vi "期末專題-記憶遊戲.vi"() -> ()   [LabVIEW 2014]
uses:
  States.ctl
  Application data.ctl
panel:
  in  "顏色順序按鈕":T1
  out "記住的顏色個數":i32
  out "顏色記憶順序":u32(colorbox)
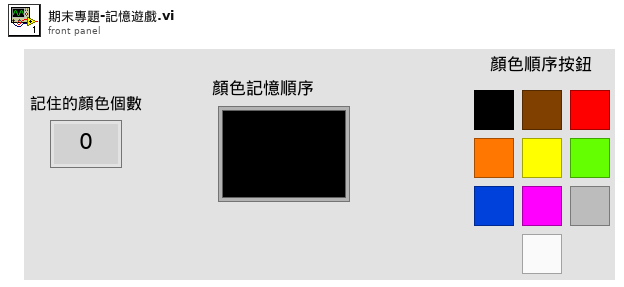
[diagram p1: front panel]
types:
  T1 = cluster{"0":bool, "7":bool, "8":bool, "9":bool, "4":bool, "5":bool, "6":bool, "1":bool, "2":bool, "3":bool}
  T2 = typedef "Application data.ctl" = cluster{"順序":i32[], "顏色":u32[], "等待時間":u32, "Last key":i16, "No.Key presses":i32, "得分":i32}
  T3 = typedef "States.ctl" = enum16{"開始", "加入新顏色", "順序", "等待", "檢查按鈕", "成功", "失敗", "結束"}
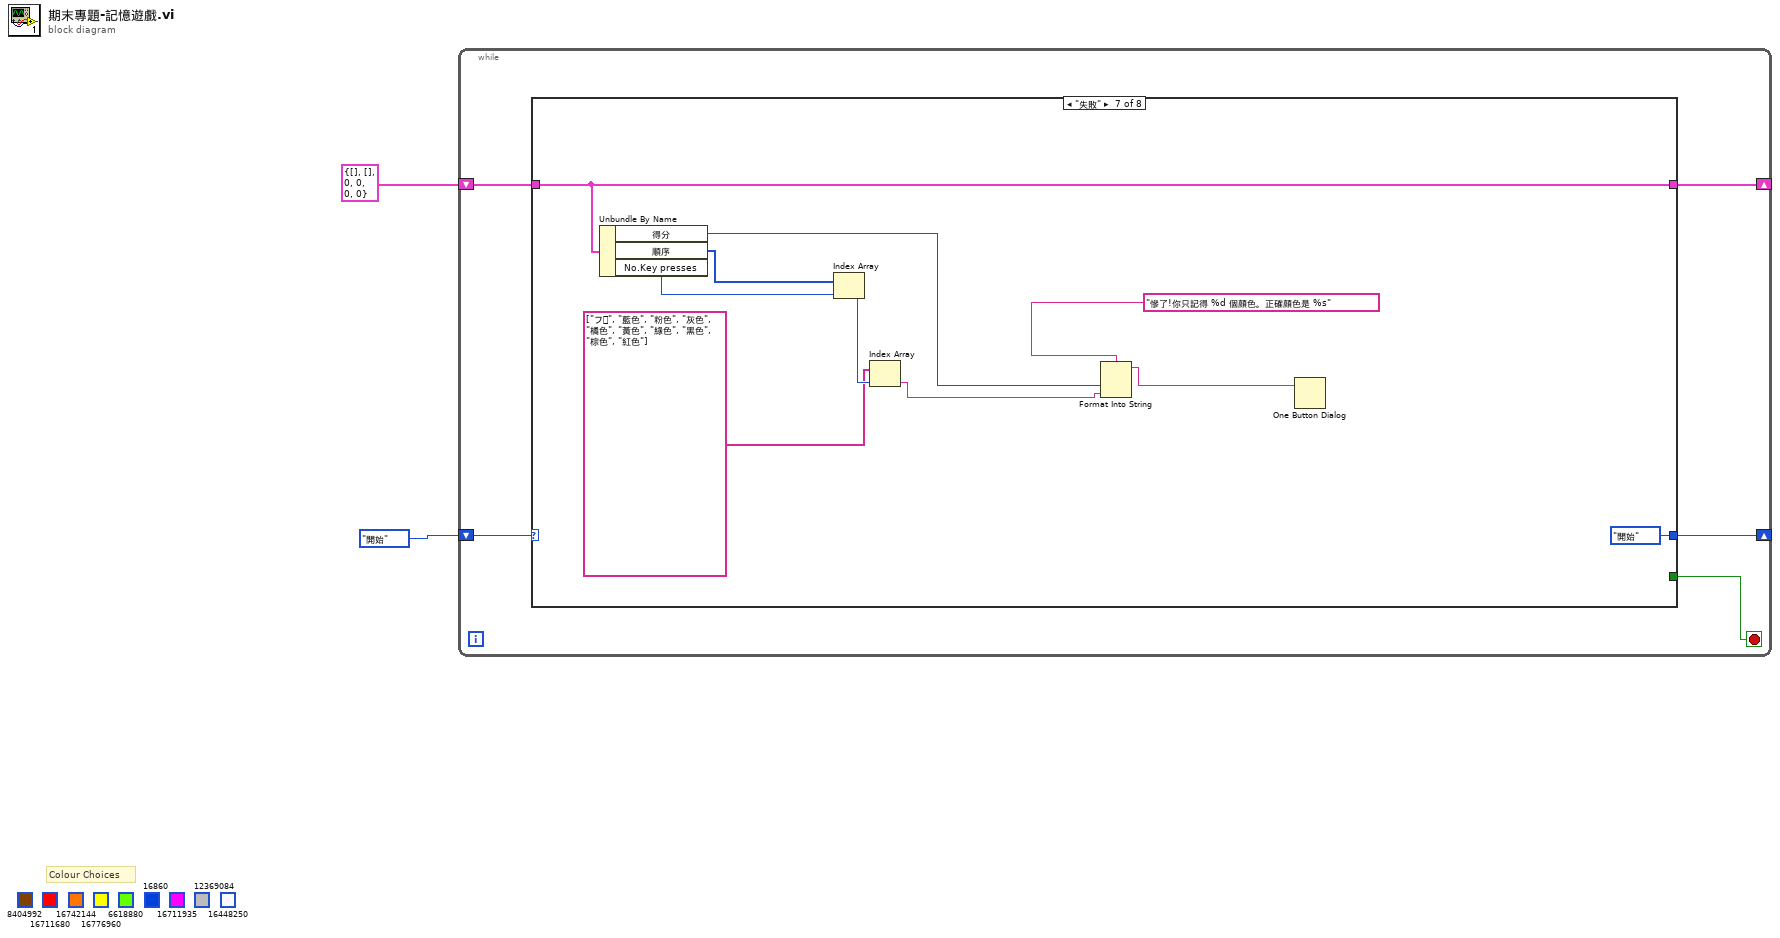
[diagram p0: block diagram]
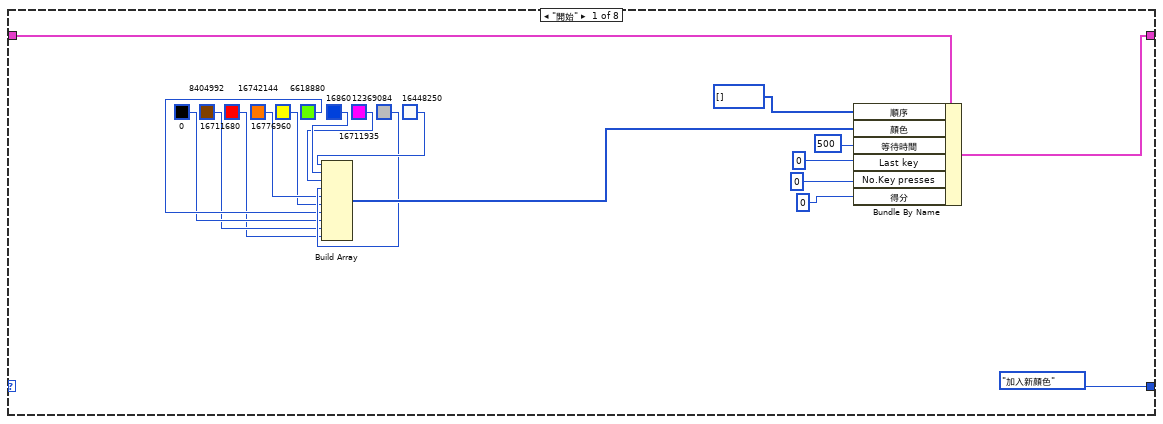
[diagram p2: hidden frame]
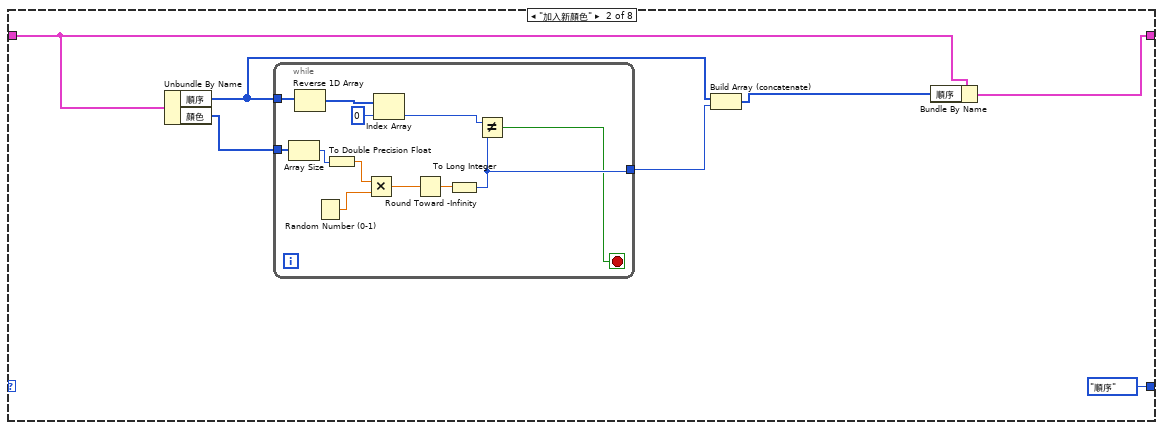
[diagram p3: hidden frame]
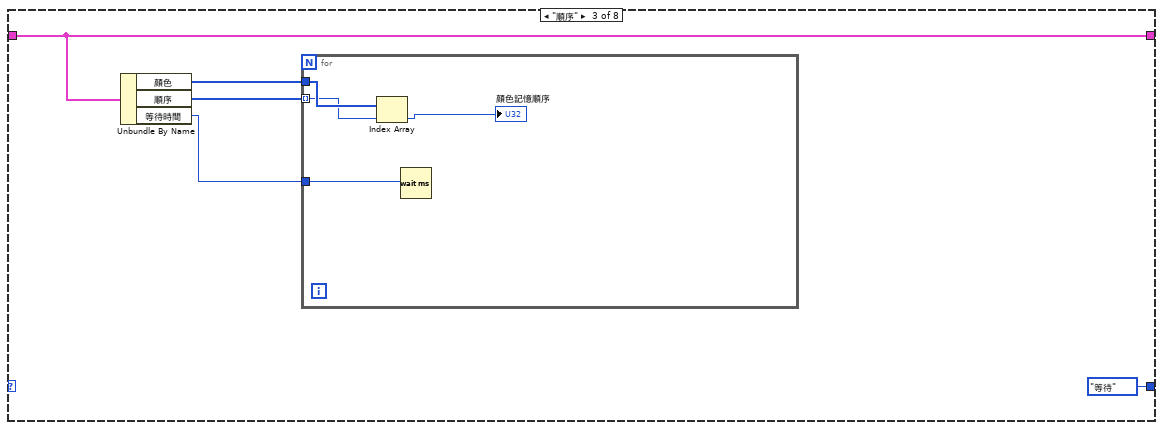
[diagram p4: hidden frame]
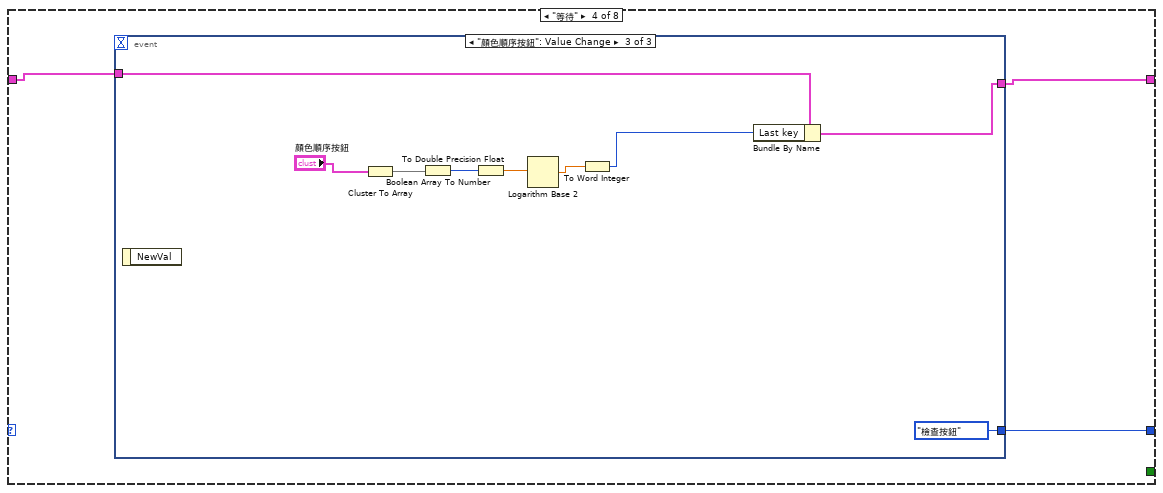
[diagram p5: hidden frame]
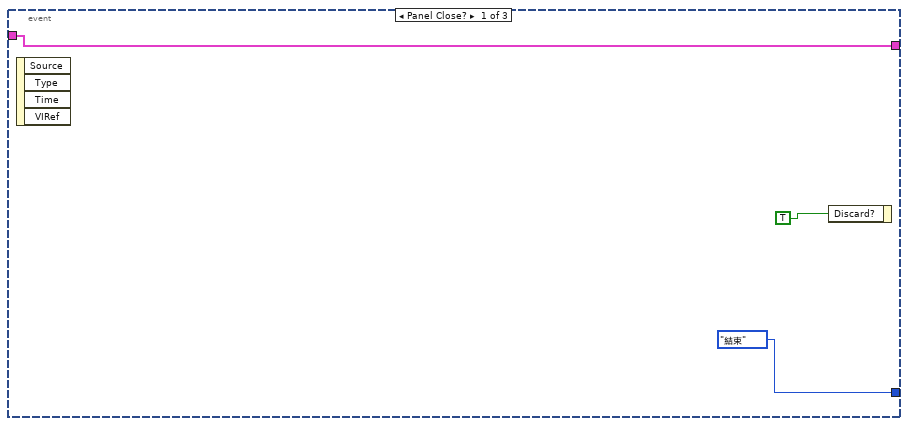
[diagram p6: hidden frame]
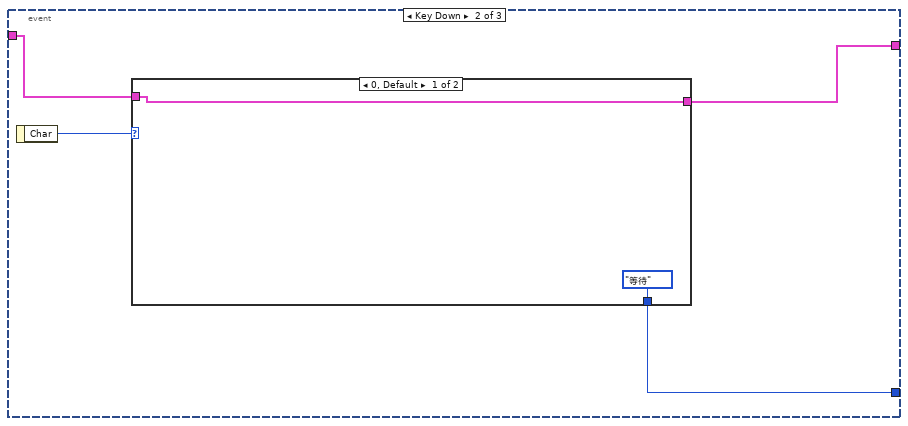
[diagram p7: hidden frame]
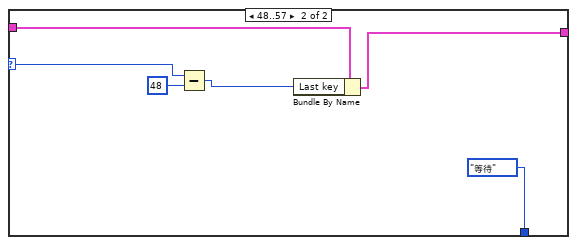
[diagram p8: hidden frame]
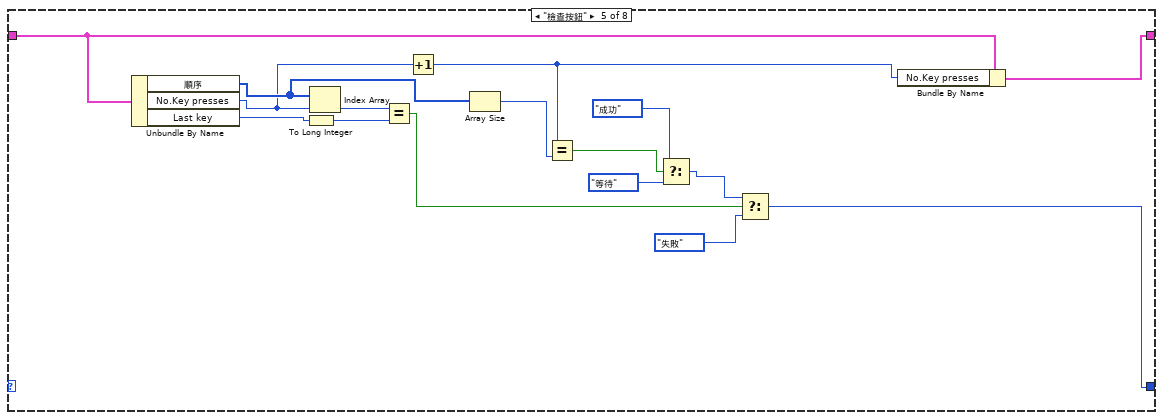
[diagram p9: hidden frame]
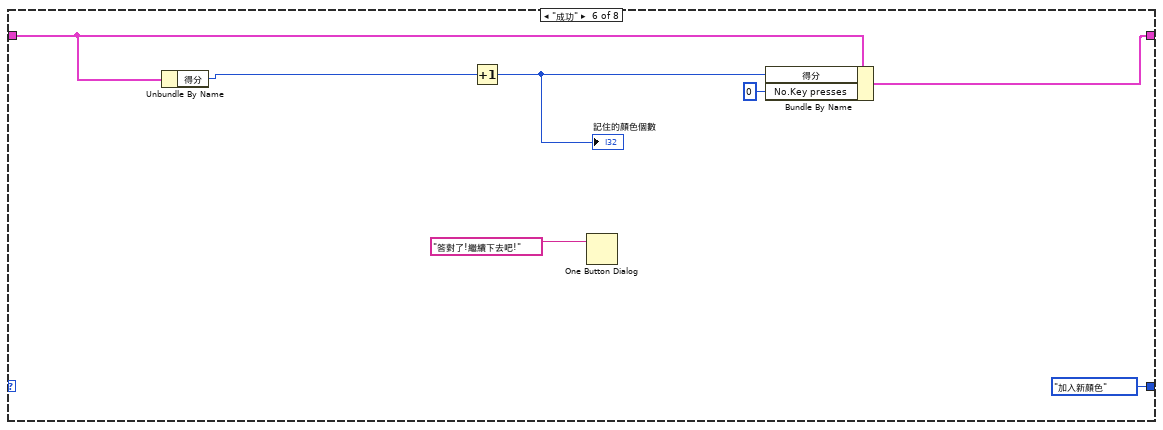
[diagram p10: hidden frame]
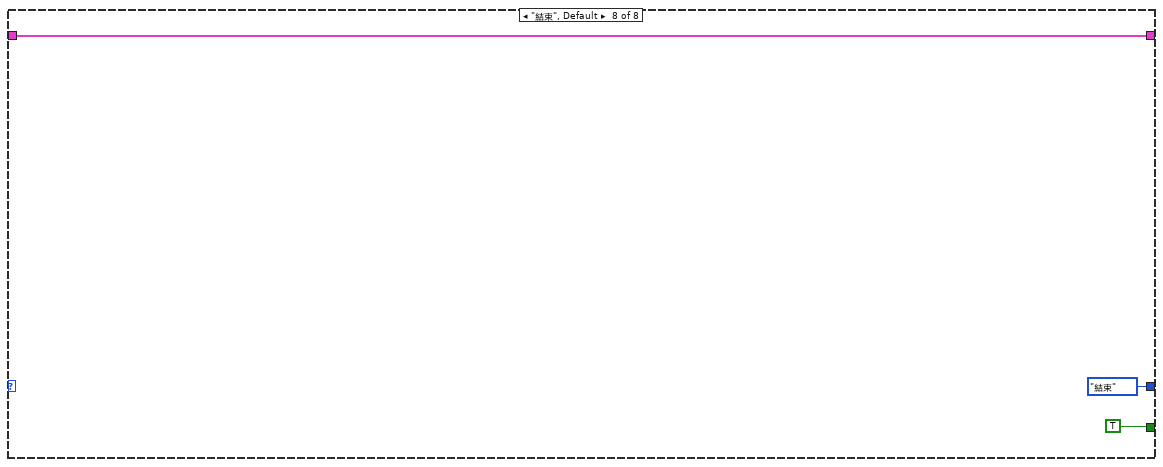
[diagram p11: hidden frame]
diagram:
  (unwired) u32 16448250 ("Color Box")
  (unwired) u32 12369084 ("Color Box")
  (unwired) u32 16711935 ("Color Box")
  (unwired) u32 16860 ("Color Box")
  (unwired) u32 6618880 ("Color Box")
  (unwired) u32 16776960 ("Color Box")
  (unwired) u32 16742144 ("Color Box")
  (unwired) u32 16711680 ("Color Box")
  (unwired) u32 8404992 ("Color Box")
  # "Colour Choices"
  n1 = while {
    shift-right: [w4] -> _
    shift-left: T2 {"順序"=[], "顏色"=[], "等待時間"=0, "Last key"=0, "No.Key presses"=0, "得分"=0} -> [w5]
    shift-right: [w3] -> _
    shift-left: States."開始" -> [w7]
    stop <- w6 stop-if-true
    n2 = case shown="\"失敗\"" w7 {
      tunnel: [_ _ _ _ _ _ _ TRUE] -> w6
      tunnel: w5 -> [w26 w30 w50 w57 w94 w103 w114 w116]
      tunnel: [w25 w28 w50 w56 w93 w102 w114 w116] -> w4
      tunnel: [States."加入新顏色" States."順序" States."等待" w55 w91 States."加入新顏色" States."開始" States."結束"] -> w3
      frame "開始" {
        n3 = Build Array(u32 16448250 ("Color Box"), u32 16860 ("Color Box"), u32 16711935 ("Color Box"), u32 12369084 ("Color Box"), u32 16742144 ("Color Box"), u32 16776960 ("Color Box"), u32 6618880 ("Color Box"), u32 0 ("Color Box"), u32 8404992 ("Color Box"), u32 16711680 ("Color Box")) -> (w19:u32[])
        n4 = Bundle By Name(cluster=w26, "順序"=i32[] [], "顏色"=w19, "等待時間"=u32 500, "Last key"=i16 0, "No.Key presses"=0, "得分"=0) -> (w25:T2)
      }
      frame "加入新顏色" {
        n5 = Unbundle By Name(w30) -> ("順序"=w32:i32[], "顏色"=w33:u32[])
        n6 = while {
          tunnel: w32 -> [w45]
          tunnel: w33 -> [w42]
          tunnel: [w35] -> w31
          stop <- w34 stop-if-true
          n7 = Array Size(array=w42) -> (size(s)=w40:i32)
          n8 = Reverse 1D Array(array=w45) -> (reversed array=w44:i32[])
          n9 = Random Number (0-1)() -> (number: 0 to 1=w43:dbl)
          n10 = To Double Precision Float(number=w40) -> (double precision float=w39:dbl)
          n11 = Multiply(x=w39, y=w43) -> (x*y=w41:dbl)
          n12 = Index Array(array=w44, index=0) -> (element=w36:i32)
          n13 = Round Toward -Infinity(1:w41) -> (0:w38:dbl)
          n14 = To Long Integer(number=w38) -> (32bit integer=w35:i32)
          n15 = Not Equal?(x=w36, y=w35) -> (x != y?=w34:bool)
        }
        n16 = Build Array (concatenate)(w32, w31) -> (w29:i32[])
        n17 = Bundle By Name(cluster=w30, "順序"=w29) -> (w28:T2)
      }
      frame "順序" {
        n18 = Unbundle By Name(w50) -> ("顏色"=w48:u32[], "順序"=w49:i32[], "等待時間"=w47:u32)
        n19 = for {
          tunnel: w49 -> [w53] mode=indexing
          tunnel: w48 -> [w54]
          tunnel: w47 -> [w51]
          n20 = Index Array(array=w54, index=w53) -> (element=→"顏色記憶順序":u32)
          n21 = Wait (ms)(milliseconds to wait=w51) -> ()  [unwired: 1 out]
        }
      }
      frame "等待" {
        n22 = event shown="[2] \"顏色順序按鈕\": Value Change" {
          selector: _ -> [_ _ _]
          dyn-events: _ -> [_ _ _]
          timeout: _ -> [_ _ _]
          tunnel: w57 -> [w60 w63 w77]
          tunnel: [w60 w62 w74] -> w56
          tunnel: [States."結束" w61 States."檢查按鈕"] -> w55
          event Panel Close? {
            n23 = event-data() -> ()  [unwired: 1 in, 4 out]
            n24 = event-data("Discard?"=TRUE) -> ()  [unwired: 1 in, 1 out]
          }
          event Key Down {
            n25 = event-data() -> ("Char"=w64:i16)  [unwired: 1 in]
            n26 = case shown="0, Default" w64 {
              selector: w64 -> [_ w69]
              tunnel: w63 -> [w66 w72]
              tunnel: [w66 w71] -> w62
              tunnel: [States."等待" States."等待"] -> w61
              frame 0, Default {
              }
              frame 48..57 {
                n27 = Subtract(x=w69, y=i16 48) -> (x-y=w68:i16)
                n28 = Bundle By Name(cluster=w72, "Last key"=w68) -> (w71:T2)
              }
            }
          }
          event "顏色順序按鈕": Value Change {
            n29 = event-data() -> ()  [unwired: 1 in, 1 out]
            n30 = Cluster To Array(cluster="顏色順序按鈕") -> (array=w80:bool[])
            n31 = Boolean Array To Number(Boolean array=w80) -> (number=w79:u32)
            n32 = To Double Precision Float(number=w79) -> (double precision float=w78:dbl)
            n33 = Logarithm Base 2(1:w78) -> (0:w76:dbl)
            n34 = To Word Integer(number=w76) -> (16bit integer=w75:i16)
            n35 = Bundle By Name(cluster=w77, "Last key"=w75) -> (w74:T2)
          }
        }
      }
      frame "檢查按鈕" {
        n36 = Unbundle By Name(w94) -> ("順序"=w85:i32[], "No.Key presses"=w83:i32, "Last key"=w96:i16)
        n37 = To Long Integer(number=w96) -> (32bit integer=w95:i32)
        n38 = Index Array(array=w85, index=w83) -> (element=w97:i32)
        n39 = Equal?(x=w97, y=w95) -> (x = y?=w92:bool)
        n40 = Increment(x=w83) -> (x+1=w82:i32)
        n41 = Array Size(array=w85) -> (size(s)=w84:i32)
        n42 = Equal?(x=w82, y=w84) -> (x = y?=w87:bool)
        n43 = Select(t=States."成功", s=w87, f=States."等待") -> (s? t:f=w89:T3)
        n44 = Select(t=w89, s=w92, f=States."失敗") -> (s? t:f=w91:T3)
        n45 = Bundle By Name(cluster=w94, "No.Key presses"=w82) -> (w93:T2)
      }
      frame "成功" {
        n46 = Unbundle By Name(w103) -> ("得分"=w99:i32)
        n47 = Increment(x=w99) -> (x+1=w98:i32)
        "記住的顏色個數" <- w98
        n48 = One Button Dialog(message="答對了!繼續下去吧!") -> ()  [unwired: 1 in, 1 out]
        n49 = Bundle By Name(cluster=w103, "得分"=w98, "No.Key presses"=0) -> (w102:T2)
      }
      frame "失敗" {
        n50 = Unbundle By Name(w114) -> ("得分"=w112:i32, "順序"=w110:i32[], "No.Key presses"=w109:i32)
        n51 = Index Array(array=w110, index=w109) -> (element=w108:i32)
        n52 = Index Array(array=string[] ["フ︹", "藍色", "粉色", "灰色", "橘色", "黃色", "綠色", "黑色", "棕色", "紅色"], index=w108) -> (element=w106:string)
        n53 = Format Into String(format string="慘了!你只記得 %d 個顏色。正確顏色是 %s" ("message"), w112, w106) -> (resulting string=w111:string)  [unwired: 2 in, 1 out]
        n54 = One Button Dialog(message=w111) -> ()  [unwired: 1 in, 1 out]
      }
      frame "結束", Default {
      }
    }
  }
